vi "SET DO AO PLC 2.vi"(10 "USCITE PLC":T1, 11 "Q":string="PLC_Q") -> ()   [LabVIEW 2019]
uses:
  Uscite PLC 2.ctl
  controls/statoAO_plc_2.ctl
  StatoDO_PLC_2.ctl
  TypeDef_PLC_Q.ctl
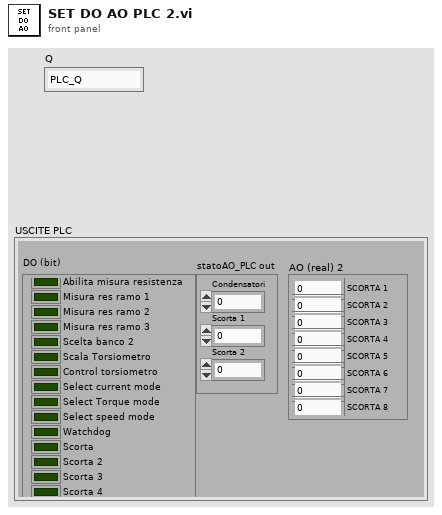
[diagram p1: front panel]
types:
  T1 = typedef "Uscite PLC 2.ctl" = cluster{"AO (real) 2":cluster{"SCORTA 1":dbl, "SCORTA 2":dbl, "SCORTA 3":dbl, "SCORTA 4":dbl, "SCORTA 5":dbl, "SCORTA 6":dbl, "SCORTA 7":dbl, "SCORTA 8":dbl}, "statoAO_PLC out":T2, "DO (bit)":T3}
  T2 = typedef "statoAO_plc_2.ctl" = cluster{"Condensatori":dbl, "Scorta 1":dbl, "Scorta 2":dbl}
  T3 = typedef "StatoDO_PLC_2.ctl" = cluster{"Relè misura resistomat":bool, "Misura res ramo 1":bool, "Misura res ramo 2":bool, "Misura res ramo 3":bool, "Scelta banco 2":bool, "Scala Torsiometro":bool, "Ctrl torsiometro":bool, "Select current mode":bool, "Select Torque mode":bool, "Select speed mode":bool, "Watchdog":bool, "Scorta":bool, "Scorta 2":bool, "Scorta 3":bool, "Scorta 4":bool, "Scorta 5":bool, "Bench selection":bool, "External alarm":bool, "Enable external program":bool, "Reset allarmi":bool, "Start":bool, "Stop":bool, "Block":bool, "Scorta 6":bool}
  T4 = typedef "TypeDef_PLC_Q.ctl" = cluster{"Message":string, "Data":variant}
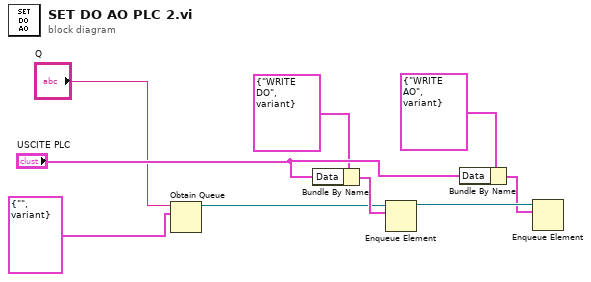
[diagram p0: block diagram]
diagram:
  n1 = Obtain Queue(name (unnamed)="Q", element data type=T4 {"Message"="", "Data"=variant}) -> (queue out=w2:refnum<queue>)  [unwired: 3 in, 2 out]
  n2 = Bundle By Name(cluster=T4 {"Message"="WRITE DO", "Data"=variant}, "Data"="USCITE PLC") -> (w4:T4)
  n3 = Enqueue Element(queue=w2, element=w4) -> (queue out=w8:refnum<queue>)  [unwired: 2 in, 2 out]
  n4 = Bundle By Name(cluster=T4 {"Message"="WRITE AO", "Data"=variant}, "Data"="USCITE PLC") -> (w7:T4)
  n5 = Enqueue Element(queue=w8, element=w7) -> ()  [unwired: 2 in, 3 out]
